vi "Detection Logic to FPGA Modularized 1Player.vi"() -> ()   [LabVIEW 2026]
uses:
  <vilib>/rvi/Emulation/niFpgaGetClockAttributes.vi
  <vilib>/rvi/Emulation/niFpgaSctlEmulationGetInTimedLoop.vi
  <vilib>/rvi/Emulation/niFpgaEmulationReportErrorSimple.vi
  <vilib>/rvi/Emulation/niFpgaEmulationIsFPGAContextNoSignature.vi
  <vilib>/rvi/errors/niFpgaSetErrorForExecOnDevCompSimple.vi
  <vilib>/rvi/eio/common/nirviEmuReportErrorAndStop.vi
  <vilib>/rvi/DataTransferAndStorage/Container/Common/niFpgaContainerGetUniqueNameForEmu.vi
  <vilib>/rvi/FIFO/Fifo_Resource/nirvififoEmulationSetSize.vi
  <vilib>/rvi/FIFO/Fifo_Resource/nirviFifoEmulationQueueMgr.vi
  <instcachedir>/0/nirviFifoEmulationQueueMgr_E5CAEC123FF24DC58D834DCA3CDAA9B5.lvgen/nirviFifoEmulationQueueMgr_E5CAEC123FF24DC58D834DCA3CDAA9B5_000.vi
  <vilib>/Utility/error.llb/Clear Errors.vi
  <vilib>/rvi/FIFO/Fifo_Resource/nirvififoEmulationCreateLock.vi
  <vilib>/rvi/Emulation/niFpgaProcessEmulError.vi
  <vilib>/rvi/FIFO/Fifo_Resource/nirvififoEmulationObtainLock.vi
  <vilib>/rvi/FIFO/Fifo_Resource/nirvififoEmulationReleaseLock.vi
  <vilib>/rvi/occurrence/nirviWaitOnOccurrenceBase.vi
  <vilib>/rvi/errors/nirviReportUnexpectedCaseInternalError.vi
  <vilib>/rvi/errors/nirviReportUnexpectedCaseInternalError (U32).vi
  <vilib>/rvi/eio/common/nirviEmuTemplateMethod_errors.vi
  <vilib>/rvi/Emulation/niFpgaCriticalErrorInLSC.vi
  <extravilib>/ChannelInstances/Tag-bool/Instantiate.vi
  <extravilib>/ChannelInstances/Tag-u8/Instantiate.vi
  <vilib>/rvi/FIFO/Fifo_Resource/nirvififoEmulationDetermineInputValidOut.vi
  <vilib>/rvi/DataTransferAndStorage/Container/XNode/niFpgaContainer.xnode
  <vilib>/rvi/FIFO/Fifo_Resource/nirvififoEmulationRead.vi
  <vilib>/eio/EIONode/EIONode.xnode
  <vilib>/rvi/FIFO/Fifo_Resource/nirvififoEmulationWrite.vi
  <instrlib>/_niInstr/Basic Elements/v1/FPGA/Private/Count Up U32.vi
  <extravilib>/ChannelInstances/Tag-bool.lvlib
  <extravilib>/ChannelInstances/Tag-u8.lvlib
  <instrlib>/_niInstr/Basic Elements/v1/FPGA/niInstr Basic Elements v1 FPGA.lvlib
panel:
  in  "Middle Lights":bool[](array[boolean])=[FALSE, FALSE, FALSE, FALSE, FALSE]
  in  "Blue-Green LEDs":u8[](array[numeric])=[0, 16, 24, 28, 30, 31] format="%.0b"
  in  "Tone length2":u32=20000
  in  "Tone length1":u32=10000
  in  "Starting Lights":bool[](array[boolean])=[FALSE, FALSE, FALSE, FALSE, FALSE, FALSE, FALSE, FALSE, FALSE, FALSE, FALSE, FALSE, FALSE, FALSE, FALSE, FALSE, FALSE, FALSE, FALSE, FALSE, FALSE, FALSE, FALSE, FALSE, FALSE, FALSE, FALSE, FALSE, FALSE, FALSE, FALSE, FALSE, FALSE, FALSE, FALSE, FALSE, FALSE, FALSE, FALSE, FALSE, FALSE, FALSE, FALSE, FALSE, FALSE]
  out "Time Remaining":u32
  in  "Game Time, uS":u32 caption="Tick Count(uSec)"
  out "Multiplier P1":u16
  out "Random Number":u8
  out "Score P1":u16
  in  "Speed Threshold, ticks":u64=3000
  in  "Debounce Threshold, ticks":u64=1000
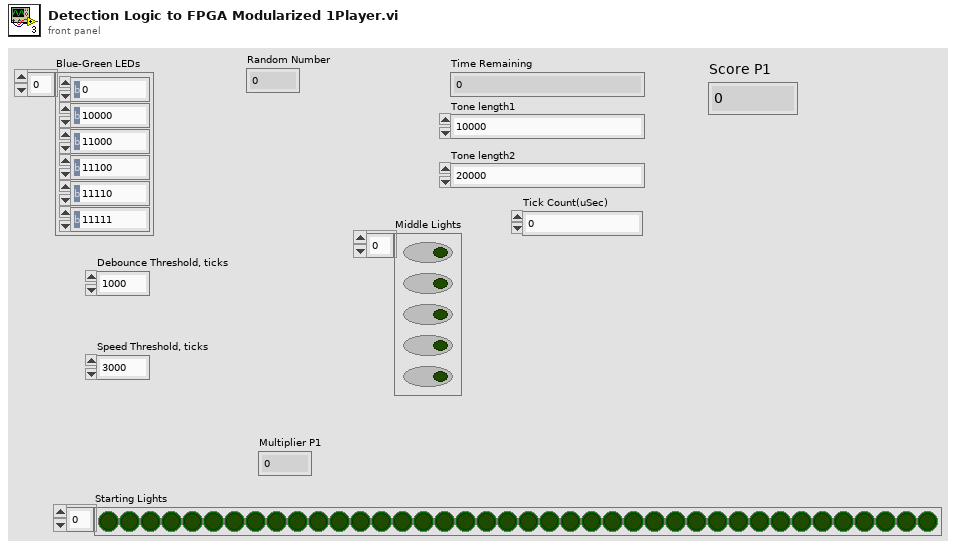
[diagram p1: front panel]
types:
  T1 = cluster{"Score":u16, "Multiplier":u16, "Last Press Tick":u64, u64[]}
  T2 = typedef "Tag-bool.lvlib/))Channel.ctl" = refnum<queue>
  T3 = cluster{"Score out":u16, "Multiplier out":u16, "Last Valid Press Tick out":u64, "Debounce Tick out":u64[]}
  T4 = typedef "Tag-u8.lvlib/))Channel.ctl" = refnum<queue>
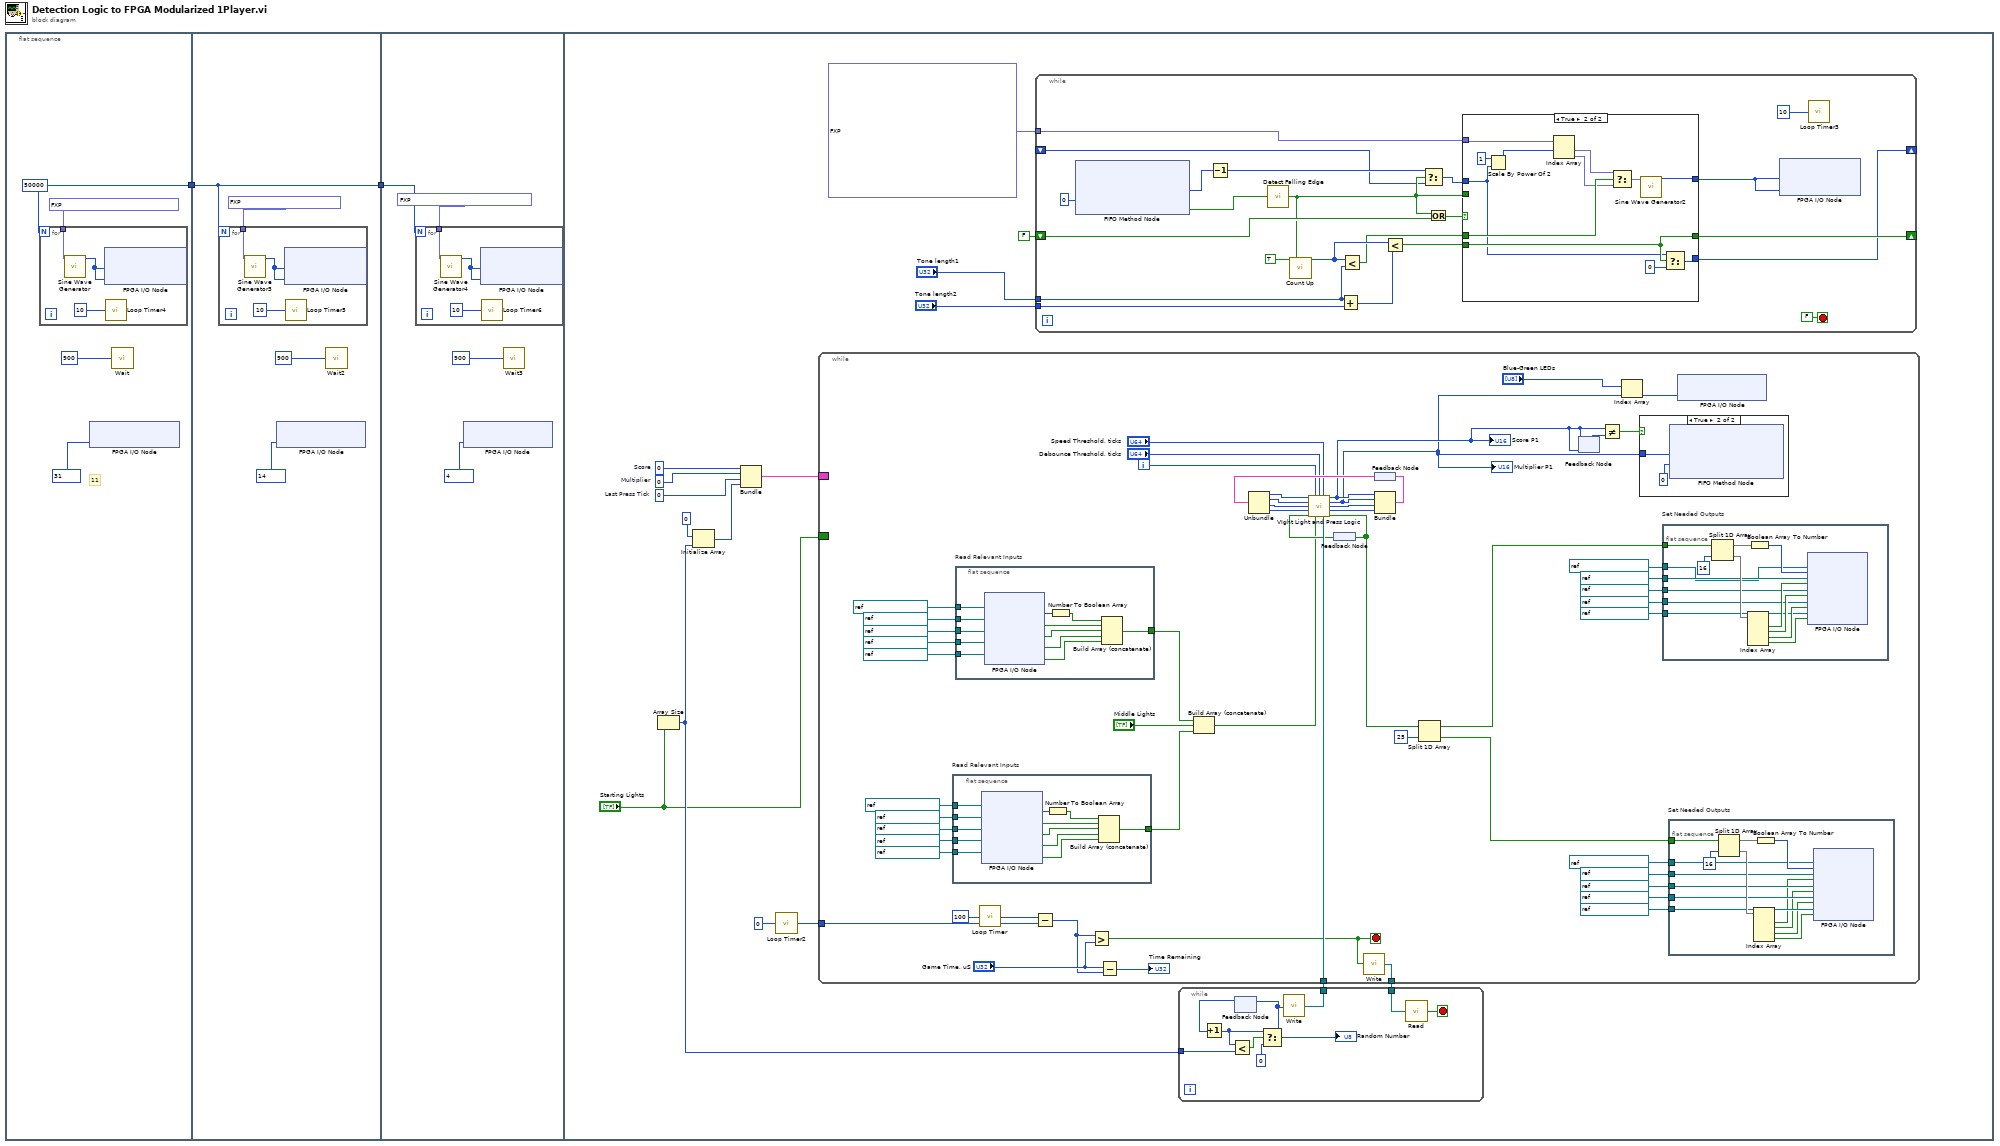
[diagram p0: block diagram]
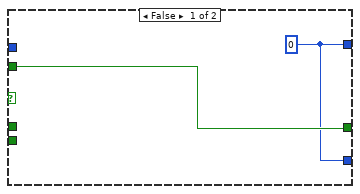
[diagram p2: hidden frame]
diagram:
  n1 = flat-sequence {
    tunnel: [w3] -> w2
    tunnel: w2 -> [w11]
    tunnel: [w11] -> w1
    tunnel: w1 -> [w18]
    frame #0 {
      w3 = 50000
      # "11"
      n2 = for {
        N: w3 -> [_]
        tunnel: fxp<+,32,0> 1.165410503745079e-05 ("frequency (periods/tick)") -> [w7]
        n3 = call "Sine Wave Generator"("frequency (periods/tick)"=w7) -> ("sine out"=w8:i16)  [unwired: 14 in]
        n4 = xnode "FPGA I/O Node"("SteroOut/AO0"=w8, "SteroOut/AO1"=w8) -> ()  [unwired: 2 in, 2 out]
        n5 = call "Loop Timer4"("Count(uSec)"=u32 10 ("Count(Ticks)")) -> ()  [unwired: 1 out]
      }
      n6 = xnode "FPGA I/O Node"("Bank-03/DO15:8"=u8 31 ("Numeric")) -> ()  [unwired: 1 in, 1 out]
      n7 = call "Wait"("Count(mSec)"=u32 900) -> ()  [unwired: 1 out]
    }
    frame #1 {
      n8 = for {
        N: w11 -> [_]
        tunnel: fxp<+,32,0> 1.8499791622161865e-05 ("frequency (periods/tick)") -> [w14]
        n9 = call "Sine Wave Generator3"("frequency (periods/tick)"=w14) -> ("sine out"=w15:i16)  [unwired: 14 in]
        n10 = xnode "FPGA I/O Node"("SteroOut/AO0"=w15, "SteroOut/AO1"=w15) -> ()  [unwired: 2 in, 2 out]
        n11 = call "Loop Timer5"("Count(uSec)"=u32 10 ("Count(Ticks)")) -> ()  [unwired: 1 out]
      }
      n12 = xnode "FPGA I/O Node"("Bank-03/DO15:8"=u8 14 ("Numeric")) -> ()  [unwired: 1 in, 1 out]
      n13 = call "Wait2"("Count(mSec)"=u32 900) -> ()  [unwired: 1 out]
    }
    frame #2 {
      n14 = for {
        N: w18 -> [_]
        tunnel: fxp<+,32,0> 2.7718255296349525e-05 ("frequency (periods/tick)") -> [w21]
        n15 = call "Sine Wave Generator4"("frequency (periods/tick)"=w21) -> ("sine out"=w22:i16)  [unwired: 14 in]
        n16 = xnode "FPGA I/O Node"("SteroOut/AO0"=w22, "SteroOut/AO1"=w22) -> ()  [unwired: 2 in, 2 out]
        n17 = call "Loop Timer6"("Count(uSec)"=u32 10 ("Count(Ticks)")) -> ()  [unwired: 1 out]
      }
      n18 = xnode "FPGA I/O Node"("Bank-03/DO15:8"=u8 4 ("Numeric")) -> ()  [unwired: 1 in, 1 out]
      n19 = call "Wait3"("Count(mSec)"=u32 900) -> ()  [unwired: 1 out]
    }
    frame #3 {
      w35 = u64 0  # Last Press Tick
      w36 = u16 0  # Multiplier
      w37 = u16 0  # Score
      n20 = Array Size(array="Starting Lights") -> (size(s)=w31:i32)
      n21 = Initialize Array(u64 0 ("Bonus Threshold"), w31) -> (w34:u64[])
      n22 = Bundle("Score"=w37, "Multiplier"=w36, "Last Press Tick"=w35, w34) -> (w33:T1)  [unwired: 1 in]
      n23 = call "Loop Timer2"("Count(uSec)"=u32 0) -> ("Tick Count(uSec)"=w29:u32)
      n24 = while {
        tunnel: fxp<+,32,0>[] [1.100008375942707e-05, 1.165410503745079e-05, 1.3081356883049011e-05, 1.3859011232852936e-05, 1.7461366951465607e-05, 1.8499791622161865e-05, 2.1999934688210487e-05, 2.330821007490158e-05, 2.6162713766098022e-05, 2.7718255296349525e-05] ("Frequency Array") -> [w49]
        shift-right: [w53] -> _
        shift-left: FALSE ("edge detected") -> [w50]
        shift-right: [w47] -> _
        shift-left: _ -> [w44]
        tunnel: "Tone length2" -> [w41]
        tunnel: "Tone length1" -> [w40]
        stop <- FALSE stop-if-true
        n25 = xnode ("FIFO Method Node")("Timeout"=0) -> ("Element"=w58:u8, "Timed Out?"=w54:bool)  [unwired: 1 in, 1 out]
        n26 = Decrement(x=w58) -> (x-1=w46:u8)
        n27 = call <instrlib>:"Detect Falling Edge.vi"("signal"=w54) -> ("edge detected"=w45:bool)  [unwired: 14 in]
        n28 = call-poly <instrlib>:"Count Up.vi"("increment"=TRUE, "reset"=w45) -> ("count out"=w57:u32)  [unwired: 13 in]
        n29 = Add(x=w40, y=w41) -> (x+y=w42:u32)
        n30 = Less?(x=w57, y=w40) -> (x < y?=w55:bool)
        n31 = Less?(x=w57, y=w42) -> (x < y?=w51:bool)
        n32 = Select(t=w46, s=w45, f=w44) -> (s? t:f=w43:i16)
        n33 = Or(x=w45, y=w50) -> (x .or. y?=w52:bool)
        n34 = case shown="True" w52 {
          tunnel: w55 -> [_ w75]
          tunnel: [w62 w73] -> w48
          tunnel: w51 -> [_ w67]
          tunnel: [w63 w67] -> w53
          tunnel: w45 -> [w63 _]
          tunnel: w49 -> [_ w70]
          tunnel: [w62 w65] -> w47
          tunnel: w43 -> [_ w64]
          frame False {
            w62 = i16 0 ("SteroOut/AO1")
          }
          frame True {
            n35 = Scale By Power Of 2(n=i16 1, x=w64) -> (x*2^n=w72:i16)
            n36 = Index Array(array=w70, index #1=w72) -> (element #1=w69:fxp<+,32,0>, element #2=w68:fxp<+,32,0>)  [unwired: 1 in]
            n37 = Select(t=w69, s=w75, f=w68) -> (s? t:f=w74:fxp<+,32,0>)
            n38 = call "Sine Wave Generator2"("frequency (periods/tick)"=w74) -> ("sine out"=w73:i16)  [unwired: 14 in]
            n39 = Select(t=w64, s=w67, f=u8 0) -> (s? t:f=w65:i16)
          }
        }
        n40 = xnode "FPGA I/O Node"("SteroOut/AO0"=w48, "SteroOut/AO1"=w48) -> ()  [unwired: 2 in, 2 out]
        n41 = call "Loop Timer3"("Count(uSec)"=u32 10 ("Count(Ticks)")) -> ()  [unwired: 1 out]
      }
      n42 = while {
        tunnel: [w129] -> w32
        border: "Starting Lights" -> [_]
        tunnel: w38 -> [w130]
        border: w33 -> [_]
        tunnel: w29 -> [w89]
        i -> [w98]
        stop <- w91 stop-if-true
        n43 = flat-sequence "Read Relevant Inputs" {
          tunnel: [w147] -> w77
          tunnel: refnum<k21> "Bank-03/DI7" ("FPGA I/O In") -> [w152]
          tunnel: refnum<k21> "Bank-03/DI6" ("FPGA I/O In") -> [w151]
          tunnel: refnum<k21> "Bank-03/DI5" ("FPGA I/O In") -> [w150]
          tunnel: refnum<k21> "Bank-03/DI4" ("FPGA I/O In") -> [w149]
          tunnel: refnum<k21> "Bank-02/DI15:0" ("FPGA I/O In") -> [w148]
          frame #0 {
            n44 = xnode "FPGA I/O Node"("FPGA I/O In"=w148, "FPGA I/O In"=w149, "FPGA I/O In"=w150, "FPGA I/O In"=w151, "FPGA I/O In"=w152) -> ("I/O Item"=w153:u16, "I/O Item"=w155:bool, "I/O Item"=w156:bool, "I/O Item"=w157:bool, "I/O Item"=w158:bool)  [unwired: 5 out]
            n45 = Number To Boolean Array(number=w153) -> (Boolean array=w154:bool[])
            n46 = Build Array (concatenate)(w154, w155, w156, w157, w158) -> (w147:bool[])
          }
        }
        n47 = flat-sequence "Read Relevant Inputs" {
          tunnel: [w178] -> w95
          tunnel: refnum<k21> "Bank-03/DI3" ("FPGA I/O In") -> [w177]
          tunnel: refnum<k21> "Bank-03/DI2" ("FPGA I/O In") -> [w176]
          tunnel: refnum<k21> "Bank-03/DI1" ("FPGA I/O In") -> [w175]
          tunnel: refnum<k21> "Bank-03/DI0" ("FPGA I/O In") -> [w174]
          tunnel: refnum<k21> "Bank-01/DI15:0" ("FPGA I/O In") -> [w173]
          frame #0 {
            n48 = xnode "FPGA I/O Node"("FPGA I/O In"=w173, "FPGA I/O In"=w174, "FPGA I/O In"=w175, "FPGA I/O In"=w176, "FPGA I/O In"=w177) -> ("I/O Item"=w179:u16, "I/O Item"=w181:bool, "I/O Item"=w182:bool, "I/O Item"=w183:bool, "I/O Item"=w184:bool)  [unwired: 5 out]
            n49 = Number To Boolean Array(number=w179) -> (Boolean array=w180:bool[])
            n50 = Build Array (concatenate)(w180, w181, w182, w183, w184) -> (w178:bool[])
          }
        }
        n51 = call "Loop Timer"("Count(uSec)"=u32 100) -> ("Tick Count(uSec)"=w86:u32)
        n52 = Subtract(x=w86, y=w89) -> (x-y=w85:u32)
        n53 = Greater?(x=w85, y="Game Time, uS") -> (0:w91:bool)
        n54 = Subtract(x="Game Time, uS", y=w85) -> (x-y=→"Time Remaining":u32)
        n55 = Build Array (concatenate)(w95, "Middle Lights", w77) -> (w94:bool[])
        n56 = feedback #1() -> (w127:bool[])
        n57 = call <extravilib>:"Write.vi"("element"=w91) -> ("channel"=w129:T2)  [unwired: 1 out]
        n58 = feedback #2() -> (w123:T1)
        n59 = Unbundle(w123) -> ("Score"=w122:u16, "Multiplier"=w121:u16, "Last Press Tick"=w120:u64, w119:u64[])
        n60 = call "VIght Light and Press Logic.vi"("Score in"=w122, "Tick"=w98, "Debounce Threshold, ticks"="Debounce Threshold, ticks", "Speed Threshold, ticks"="Speed Threshold, ticks", "Multiplier in"=w121, "Last Valid Press Tick in"=w120, "Debounce Tick in"=w119, "Lit Buttons"=w127, "Pressed Buttons"=w94, "Random Number"=w130) -> ("Score out"=w83:u16, "Multiplier out"=w79:u16, "Last Valid Press Tick out"=w125:u64, "Debounce Tick out"=w126:u64[], "Buttons to Light"=w92:bool[])  [unwired: 1 in]
        "Score P1" <- w83
        "Multiplier P1" <- w79
        n61 = feedback-in #1(w92) -> ()
        n62 = Bundle("Score out"=w83, "Multiplier out"=w79, "Last Valid Press Tick out"=w125, "Debounce Tick out"=w126) -> (w124:T3)  [unwired: 1 in]
        n63 = feedback-in #2(w124) -> ()
        n64 = Split 1D Array(array=w92, index=25) -> (first subarray=w90:bool[], second subarray=w78:bool[])
        n65 = feedback-in #3(w83) -> ()
        n66 = feedback #3(w83) -> (w84:u16)
        n67 = Not Equal?(x=w83, y=w84) -> (x != y?=w82:bool)
        n68 = Index Array(array="Blue-Green LEDs", index=w79) -> (element=w80:u8)
        n69 = case shown="True" w82 {
          tunnel: w79 -> [_ w131]
          frame False {
          }
          frame True {
            n70 = xnode ("FIFO Method Node")("Element"=w131, "Timeout"=0) -> ()  [unwired: 1 in, 2 out]
          }
        }
        n71 = flat-sequence "Set Needed Outputs" {
          tunnel: w90 -> [w172]
          tunnel: refnum<k21> "Bank-03/DO3" ("FPGA I/O In") -> [w159]
          tunnel: refnum<k21> "Bank-03/DO2" ("FPGA I/O In") -> [w163]
          tunnel: refnum<k21> "Bank-03/DO1" ("FPGA I/O In") -> [w162]
          tunnel: refnum<k21> "Bank-03/DO0" ("FPGA I/O In") -> [w161]
          tunnel: refnum<k21> "Bank-01/DO15:0" ("FPGA I/O In") -> [w160]
          frame #0 {
            n72 = Split 1D Array(array=w172, index=16) -> (first subarray=w170:bool[], second subarray=w168:bool[])
            n73 = Index Array(array=w168) -> (element #1=w167:bool, element #2=w166:bool, element #3=w165:bool, element #4=w164:bool)  [unwired: 4 in]
            n74 = Boolean Array To Number(Boolean array=w170) -> (number=w171:u32)
            n75 = xnode "FPGA I/O Node"("I/O Item"=w171, "FPGA I/O In"=w160, "I/O Item"=w167, "FPGA I/O In"=w161, "I/O Item"=w166, "FPGA I/O In"=w162, "I/O Item"=w165, "FPGA I/O In"=w163, "I/O Item"=w164, "FPGA I/O In"=w159) -> ()  [unwired: 5 out]
          }
        }
        n76 = flat-sequence "Set Needed Outputs" {
          tunnel: refnum<k21> "Bank-03/DO7" ("FPGA I/O In") -> [w140]
          tunnel: refnum<k21> "Bank-03/DO6" ("FPGA I/O In") -> [w143]
          tunnel: refnum<k21> "Bank-03/DO5" ("FPGA I/O In") -> [w142]
          tunnel: refnum<k21> "Bank-03/DO4" ("FPGA I/O In") -> [w141]
          tunnel: refnum<k21> "Bank-02/DO15:0" ("FPGA I/O In") -> [w138]
          tunnel: w78 -> [w139]
          frame #0 {
            n77 = Split 1D Array(array=w139, index=16) -> (first subarray=w137:bool[], second subarray=w144:bool[])
            n78 = Index Array(array=w144) -> (element #1=w136:bool, element #2=w135:bool, element #3=w134:bool, element #4=w133:bool)  [unwired: 4 in]
            n79 = Boolean Array To Number(Boolean array=w137) -> (number=w146:u32)
            n80 = xnode "FPGA I/O Node"("I/O Item"=w146, "FPGA I/O In"=w138, "I/O Item"=w136, "FPGA I/O In"=w141, "I/O Item"=w135, "FPGA I/O In"=w142, "I/O Item"=w134, "FPGA I/O In"=w143, "I/O Item"=w133, "FPGA I/O In"=w140) -> ()  [unwired: 5 out]
          }
        }
        n81 = xnode "FPGA I/O Node"("Bank-03/DO15:8"=w80) -> ()  [unwired: 1 in, 1 out]
      }
      n82 = while {
        tunnel: w32 -> [w189]
        tunnel: w31 -> [w186]
        tunnel: [w185] -> w38
        stop <- w188 stop-if-true
        n83 = feedback #4() -> (w191:u8)  [unwired: 1 in]
        n84 = Increment(x=w191) -> (x+1=w187:u8)
        n85 = Less?(x=w187, y=w186) -> (x < y?=w192:bool)
        n86 = Select(t=w187, s=w192, f=u8 0) -> (s? t:f=w193:u8)
        "Random Number" <- w193
        n87 = feedback-in #4(w193) -> ()
        n88 = call <extravilib>:"Write.vi"("element"=w193) -> ("channel"=w185:T4)  [unwired: 1 out]
        n89 = call <extravilib>:"Read.vi"("channel"=w189) -> ("element"=w188:bool)  [unwired: 1 in, 1 out]
      }
    }
  }
